vi "VariantToType.vi"(11 "Variant":variant) -> (3 "type Name":string)   [LabVIEW 2020]
uses:
  <vilib>/Utility/VariantDataType/VariantType.lvlib
  <vilib>/Utility/Data Type/NI_Data Type.lvlib
panel:
  # "Get Types of variant"
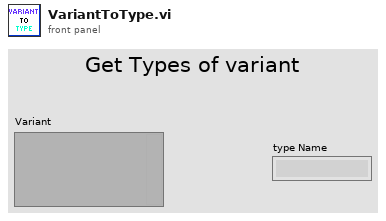
[diagram p1: front panel]
types:
  T1 = typedef "NI_Data Type.lvlib/Data Type.ctl" = enum8{"Invalid Type", "Void", "I8", "I16", "I32", "I64", "U8", "U16", "U32", "U64", "Single Float", "Double Float", "Extended Float", "Single Complex", "Double Complex", "Extended Complex", "Enum U8", "Enum U16", "Enum U32", "Enum U64", "Single Float With Unit", "Double Float With Unit", "Extended Float With Unit", "Single Complex with Unit", "Double Complex with Unit", "Extended Complex with Unit", "Boolean", "String", "Path", "Picture", "Tag", "Array", "Cluster", "Variant", "LV Variant", "Waveform", "Timestamp", "Digital Waveform", "Digital Data", "ExpressData", "Refnum", "External Data", "VI", "Poly VI", "LabVIEW Class Instance", "Fixed Point", "Set Collection", "Map Collection"}
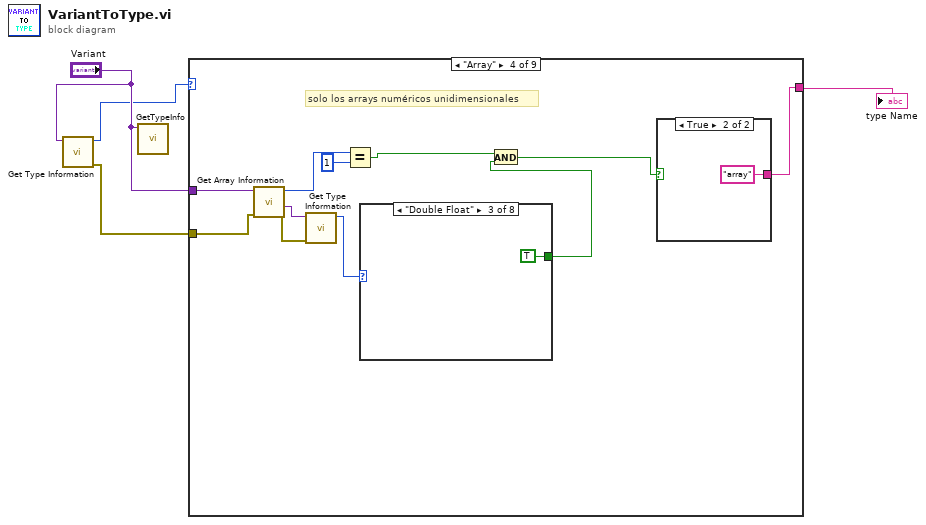
[diagram p0: block diagram]
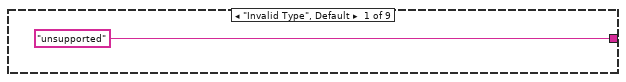
[diagram p2: hidden frame]
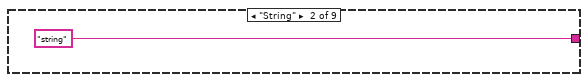
[diagram p3: hidden frame]
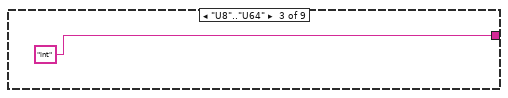
[diagram p4: hidden frame]
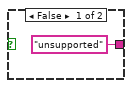
[diagram p5: hidden frame]
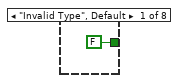
[diagram p6: hidden frame]
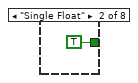
[diagram p7: hidden frame]
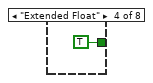
[diagram p8: hidden frame]
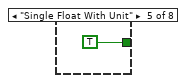
[diagram p9: hidden frame]
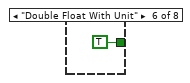
[diagram p10: hidden frame]
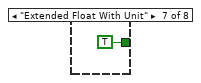
[diagram p11: hidden frame]
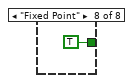
[diagram p12: hidden frame]
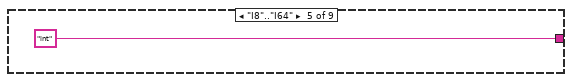
[diagram p13: hidden frame]
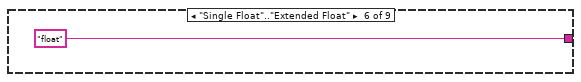
[diagram p14: hidden frame]
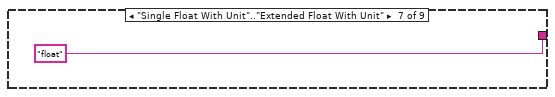
[diagram p15: hidden frame]
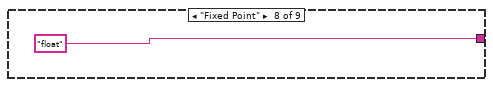
[diagram p16: hidden frame]
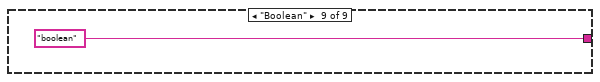
[diagram p17: hidden frame]
diagram:
  n1 = call <vilib>:"Get Type Information.vi"("variant"="Variant") -> ("error out"=w1:errorcluster, "type"=w2:T1)  [unwired: 6 in, 3 out]
  n2 = call <vilib>:"GetTypeInfo.vi"("Variant"="Variant") -> ()  [unwired: 6 in, 5 out]
  n3 = case shown="\"Array\"" w2 {
    tunnel: ["unsupported" "string" "int" w8 "int" "float" "float" "float" "boolean"] -> w4
    tunnel: "Variant" -> [_ _ _ w18 _ _ _ _ _]
    tunnel: w1 -> [_ _ _ w14 _ _ _ _ _]
    frame "Invalid Type", Default {
    }
    frame "String" {
    }
    frame "U8".."U64" {
    }
    frame "Array" {
      # "solo los arrays numéricos unidimensionales"
      n4 = call <vilib>:"Get Array Information.vi"("error in (no error)"=w14, "variant"=w18) -> ("error out"=w13:errorcluster, "array element data type"=w15:variant, "number of dimensions"=w17:i32)  [unwired: 6 in, 1 out]
      n5 = call <vilib>:"Get Type Information.vi"("error in (no error)"=w13, "variant"=w15) -> ("type"=w12:T1)  [unwired: 5 in, 4 out]
      n6 = Equal?(x=w17, y=1) -> (x = y?=w11:bool)
      n7 = case shown="\"Double Float\"" w12 {
        tunnel: [FALSE ("y") TRUE ("y") TRUE ("y") TRUE ("y") TRUE ("y") TRUE ("y") TRUE ("y") TRUE ("y")] -> w10
        frame "Invalid Type", Default {
        }
        frame "Single Float" {
        }
        frame "Double Float" {
        }
        frame "Extended Float" {
        }
        frame "Single Float With Unit" {
        }
        frame "Double Float With Unit" {
        }
        frame "Extended Float With Unit" {
        }
        frame "Fixed Point" {
        }
      }
      n8 = And(x=w11, y=w10) -> (x .and. y?=w9:bool)
      n9 = case shown="True" w9 {
        tunnel: ["unsupported" "array"] -> w8
        frame False {
        }
        frame True {
        }
      }
    }
    frame "I8".."I64" {
    }
    frame "Single Float".."Extended Float" {
    }
    frame "Single Float With Unit".."Extended Float With Unit" {
    }
    frame "Fixed Point" {
    }
    frame "Boolean" {
    }
  }
  "type Name" <- w4
